vi "PulseOut.vi"(8 "error in (no error)":errorcluster, 11 "reference":refnum<k24>) -> (0 "error out":errorcluster, 1 "LowTicks":u32, 2 "HighTicks":u32, 3 "reference out":refnum<k24>, 4 "LowTime":dbl, 5 "Frequency":dbl, 6 "HighTime":dbl, 7 "DutyCycle":dbl)   [LabVIEW 2009]
uses:
  C:/Program Files/National Instruments/LabVIEW 2009/vi.lib/ULx/ULx_LV.dll
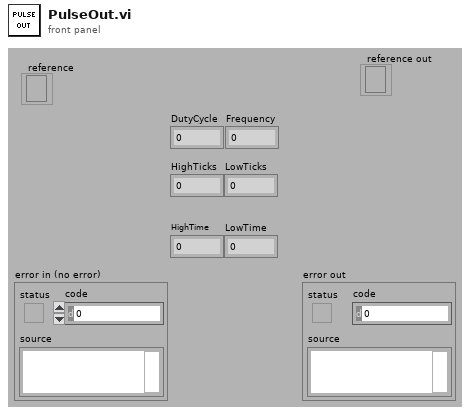
[diagram p1: front panel]
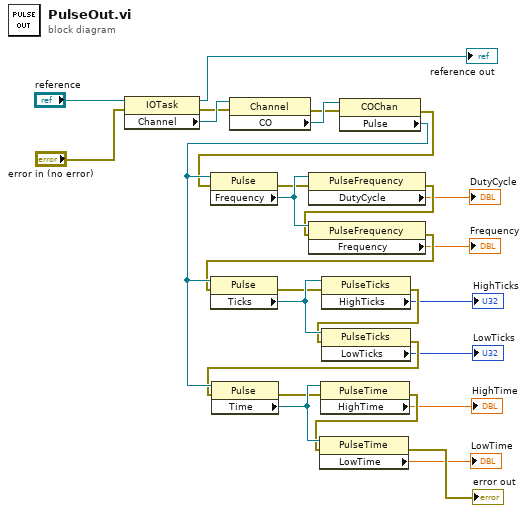
[diagram p0: block diagram]
diagram:
  n1 = property class="IOTask"(reference="reference", error in="error in (no error)") -> (reference out=→"reference out":refnum<k24>, error out=w22:errorcluster, "Channel"=w27:refnum<k24>)
  n2 = property class="Channel"(reference=w27, error in=w22) -> (error out=w21:errorcluster, "CO"=w26:refnum<k24>)  [unwired: 1 out]
  n3 = property class="COChan"(reference=w26, error in=w21) -> (error out=w19:errorcluster, "Pulse"=w20:refnum<k24>)  [unwired: 1 out]
  n4 = property class="Pulse"(reference=w20, error in=w19) -> (error out=w17:errorcluster, "Frequency"=w18:refnum<k24>)  [unwired: 1 out]
  n5 = property class="PulseFrequency"(reference=w18, error in=w17) -> (error out=w16:errorcluster, "DutyCycle"=→"DutyCycle":dbl)  [unwired: 1 out]
  n6 = property class="PulseFrequency"(reference=w18, error in=w16) -> (error out=w15:errorcluster, "Frequency"=→"Frequency":dbl)  [unwired: 1 out]
  n7 = property class="Pulse"(reference=w20, error in=w15) -> (error out=w13:errorcluster, "Ticks"=w14:refnum<k24>)  [unwired: 1 out]
  n8 = property class="PulseTicks"(reference=w14, error in=w13) -> (error out=w12:errorcluster, "HighTicks"=→"HighTicks":u32)  [unwired: 1 out]
  n9 = property class="PulseTicks"(reference=w14, error in=w12) -> (error out=w11:errorcluster, "LowTicks"=→"LowTicks":u32)  [unwired: 1 out]
  n10 = property class="Pulse"(reference=w20, error in=w11) -> (error out=w9:errorcluster, "Time"=w10:refnum<k24>)  [unwired: 1 out]
  n11 = property class="PulseTime"(reference=w10, error in=w9) -> (error out=w8:errorcluster, "HighTime"=→"HighTime":dbl)  [unwired: 1 out]
  n12 = property class="PulseTime"(reference=w10, error in=w8) -> (error out=→"error out":errorcluster, "LowTime"=→"LowTime":dbl)  [unwired: 1 out]
